vi "SubVI_Read_PHD_FromTXT_ver2.4.vi"(7 "file path (dialog if empty)":path) -> (3 "PHDValues":dbl[](array[numeric]))   [LabVIEW 2018]
uses:
  <vilib>/Utility/file.llb/Read Delimited Spreadsheet (DBL).vi
panel:
  out "all rows":dbl[][](array[numeric])
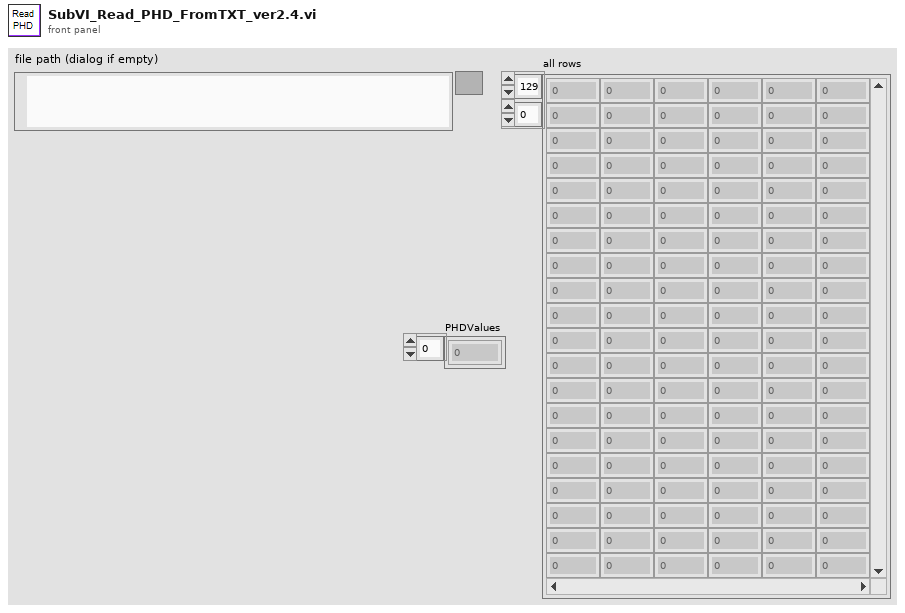
[diagram p1: front panel]
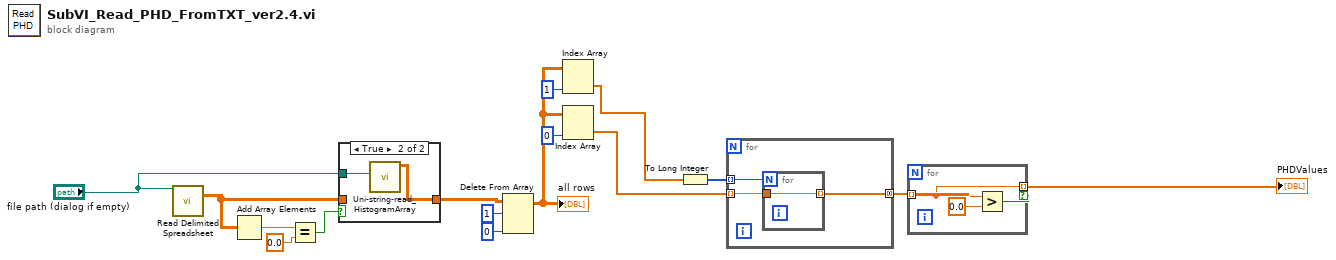
[diagram p0: block diagram]
diagram:
  n1 = call-poly <vilib>:"Read Delimited Spreadsheet.vi"("file path (dialog if empty)"="file path (dialog if empty)") -> ("all rows"=w4:dbl[][])  [unwired: 9 in, 5 out]
  n2 = Add Array Elements(numeric array=w4) -> (sum=w7:dbl)
  n3 = Equal?(x=w7, y=0.0) -> (x = y?=w5:bool)
  n4 = case shown="True" w5 {
    tunnel: "file path (dialog if empty)" -> [_ w19]
    tunnel: w4 -> [w17 _]
    tunnel: [w17 w18] -> w3
    frame False {
    }
    frame True {
      n5 = call "Uni-string-read_HistogramArray.vi"("file (use dialog)"=w19) -> ("Histogram Array"=w18:dbl[][])  [unwired: 4 in, 6 out]
    }
  }
  n6 = Delete From Array(array=w3, length=1, index (row)=0) -> (array with subset deleted=w13:dbl[][])  [unwired: 1 in, 1 out]
  "all rows" <- w13
  n7 = Index Array(array=w13, index (col)=1 ("disabled index (col)")) -> (element=w9:dbl[])  [unwired: 1 in]
  n8 = Index Array(array=w13, index (col)=0 ("disabled index (col)")) -> (element=w11:dbl[])  [unwired: 1 in]
  n9 = To Long Integer(number=w9) -> (32bit integer=w10:i32[])
  n10 = for {
    tunnel: w11 -> [w22] mode=indexing
    tunnel: w10 -> [w21] mode=indexing
    tunnel: [w20] -> w8 mode=concatenating
    n11 = for {
      N: w21 -> [_]
      tunnel: w22 -> [w23]
      tunnel: [w23] -> w20 mode=indexing
    }
  }
  n12 = for {
    tunnel: w8 -> [w25] mode=indexing
    tunnel: [w25] -> w2 mode=indexing if=w24
    n13 = Greater?(x=w25, y=0.0) -> (0:w24:bool)
  }
  "PHDValues" <- w2
